vi "IPtoInt (SubVI).vi"(11 "IP_PC":string) -> (3 "Numeric":u32 format="%x")   [LabVIEW 2017]
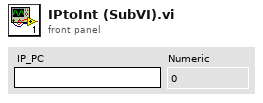
[diagram p1: front panel]
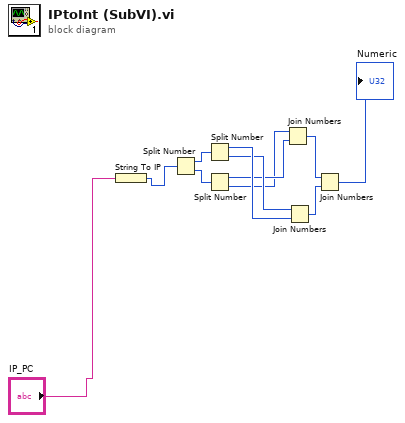
[diagram p0: block diagram]
diagram:
  n1 = String To IP(1:"IP_PC") -> (0:w10:u32)
  n2 = Split Number(x=w10) -> (hi(x)=w1:u16, lo(x)=w2:u16)
  n3 = Split Number(x=w1) -> (hi(x)=w6:u8, lo(x)=w5:u8)
  n4 = Split Number(x=w2) -> (hi(x)=w4:u8, lo(x)=w3:u8)
  n5 = Join Numbers(hi=w3, lo=w4) -> ((hi.lo)=w7:u16)
  n6 = Join Numbers(hi=w5, lo=w6) -> ((hi.lo)=w8:u16)
  n7 = Join Numbers(hi=w7, lo=w8) -> ((hi.lo)=→"Numeric":u32)
